vi "Digital_Write.vi"(8 "error in (no error)":errorcluster, 9 "Pin":u8=4 min=4 max=40, 10 "Estado":bool, 11 "VISA resource name":refnum<visa-resource-name>) -> (0 "error out":errorcluster, 3 "VISA resource name out":refnum<visa-resource-name>)   [LabVIEW 2025]
doc: "Este VI permite enviar una instruccion de escritura digital al pin elegido asi como su estado logico \nDebe recibir los datos de VISA resource name, Error IN, el pin y estado logico\nDara como salida VISA resource name y error OUT"
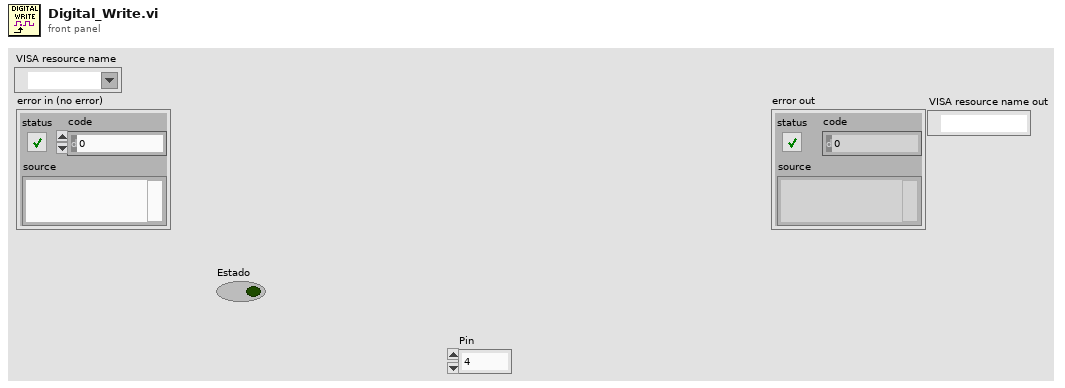
[diagram p1: front panel]
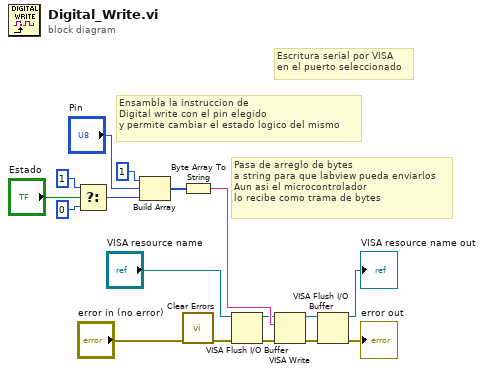
[diagram p0: block diagram]
diagram:
  # "Escritura serial por VISA\nen el puerto seleccionado"
  # "Pasa de arreglo de bytes \na string para que labview pueda enviarlos\nAun asi el microcontrolador\nlo recibe como trama de bytes"
  # "Ensambla la instruccion de \nDigital write con el pin elegido\ny permite cambiar el estado logico del mismo"
  n1 = Select(t=u8 1, s="Estado", f=u8 0) -> (s? t:f=w10:u8)
  n2 = Build Array(u8 1, "Pin", w10) -> (w15:u8[])
  n3 = Byte Array To String(unsigned byte array=w15) -> (string=w17:string)
  n4 = call <vilib>:"Clear Errors.vi"("error in (no error)"="error in (no error)") -> ("error out"=w1:errorcluster)  [unwired: 5 in, 1 out]
  n5 = VISA Flush I/O Buffer(VISA resource name="VISA resource name", error in (no error)=w1) -> (VISA resource name out=w3:refnum<visa-resource-name>, error out=w4:errorcluster)  [unwired: 1 in]
  n6 = VISA Write(VISA resource name=w3, write buffer=w17, error in (no error)=w4) -> (VISA resource name out=w5:refnum<visa-resource-name>, error out=w8:errorcluster)  [unwired: 1 out]
  n7 = VISA Flush I/O Buffer(VISA resource name=w5, error in (no error)=w8) -> (VISA resource name out=→"VISA resource name out":refnum<visa-resource-name>, error out=→"error out":errorcluster)  [unwired: 1 in]
